vi "getRobotModelStateSpace.vi"(8 "error in (no error)":errorcluster, 10 "StateSpaceTestParameters":T1, 11 "Game in":refnum<class "Game.lvclass">) -> (0 "error out":errorcluster, 1 "State":T2 {"progress" scale=0.0..100.0}, 2 "TestTeam":refnum<class "Ally.lvclass">, 3 "Game out":refnum<class "Game.lvclass">)   [LabVIEW 2021, in "Game.lvclass"]
uses:
  Game.lvclass
  Controls/RobotModelTestState.ctl
  Ally_class/Ally.lvclass
  D:/RoboIme/controle/SSL_AI/Team_class/Team.lvclass
  Game.lvclass/Game.ctl
  Team_class/Team.lvclass/Team.ctl
  Robot_class/Robot.lvclass/Robot.ctl
  <vilib>/Analysis/coordinate.llb/2D Cartesian Coordinate Rotation (Scalar).vi
  Read TestTeam.vi
  Read AllyRef.vi
  Team_class/Read RobotRef.vi
  Robot_class/Read orientation.vi
  Robot_class/Write v_tang.vi
  Robot_class/Write v_norm.vi
  Robot_class/Write v_ang.vi
  Team_class/Write RobotRef.vi
  Robot_class/Robot.lvclass
  Utilities_class/Utilities.lvclass
  <vilib>/Analysis/NI_AALPro.lvlib
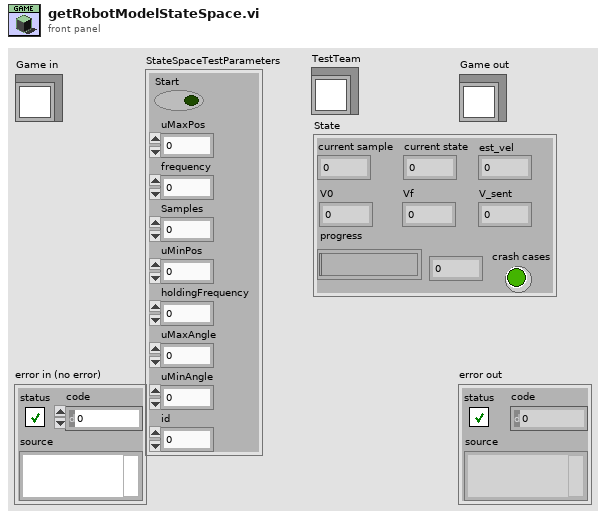
[diagram p1: front panel]
types:
  T1 = cluster{"Start":bool, "uMaxPos":dbl, "frequency":i32, "Samples":dbl, "uMinPos":dbl, "holdingFrequency":dbl, "uMaxAngle":dbl, "uMinAngle":dbl, "id":dbl}
  T2 = typedef "RobotModelTestState.ctl" = cluster{"current sample":i32, "V0":dbl, "Vf":dbl, "progress":dbl, "current state":i32, "est_vel":dbl, "V_sent":dbl, "crash cases":bool}
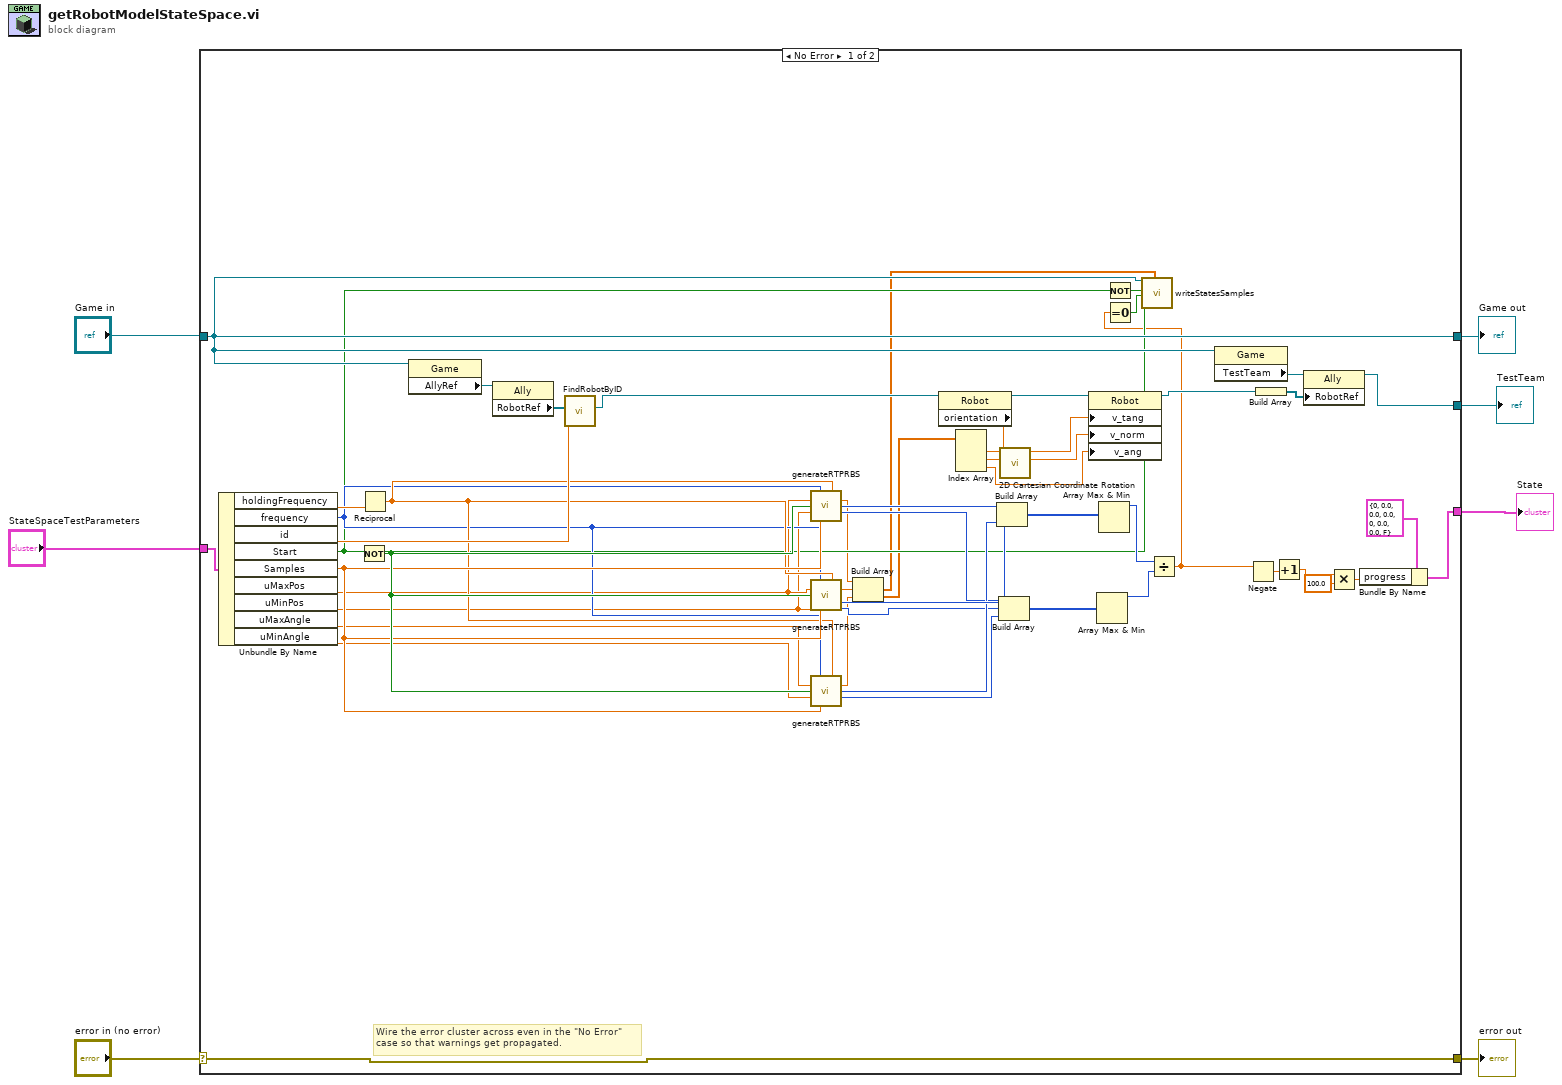
[diagram p0: block diagram]
diagram:
  n1 = case shown="No Error" "error in (no error)" {
    selector: "error in (no error)" -> [w58 w60]
    tunnel: [w58 w60] -> w6
    tunnel: [w21 w59] -> w4
    tunnel: "Game in" -> [w21 w59]
    tunnel: "StateSpaceTestParameters" -> [w55 _]
    tunnel: [w51 _] -> w3
    tunnel: [w49 _] -> w2
    frame No Error {
      # "Wire the error cluster across even in the \"No Error\"\ncase so that warnings get propagated."
      n2 = Unbundle By Name(w55) -> ("holdingFrequency"=w42:dbl, "frequency"=w40:i32, "id"=w54:dbl, "Start"=w19:bool, "Samples"=w43:dbl, "uMaxPos"=w39:dbl, "uMinPos"=w38:dbl, "uMaxAngle"=w37:dbl, "uMinAngle"=w36:dbl)
      n3 = Not(x=w19) -> (.not. x?=w44:bool)
      n4 = Reciprocal(x=w42) -> (1/x=w41:dbl)
      n5 = property class="Game"(reference=w21) -> ("AllyRef"=w57:refnum<class "Ally.lvclass">)  [unwired: 1 in, 2 out]
      n6 = property class="Ally"(reference=w57) -> ("RobotRef"=w56:refnum<class "Robot.lvclass">[])  [unwired: 1 in, 2 out]
      n7 = call "FindRobotByID.vi"("id"=w54, "RobotRef"=w56) -> ("Robot"=w48:refnum<class "Robot.lvclass">)  [unwired: 6 in, 3 out]
      n8 = call "generateRTPRBS.vi"("W"=w40, "Th"=w41, "MAX"=w39, "activate"=w44, "MIN"=w38, "PRBS samples"=w43) -> ("Val"=w18:dbl, "Size"=w35:i32, "totalSize"=w32:i32)  [unwired: 5 in, 2 out]
      n9 = call "generateRTPRBS.vi"("W"=w40, "Th"=w41, "MAX"=w39, "activate"=w44, "MIN"=w38, "PRBS samples"=w43) -> ("Val"=w17:dbl, "Size"=w34:i32, "totalSize"=w31:i32)  [unwired: 5 in, 2 out]
      n10 = call "generateRTPRBS.vi"("W"=w40, "Th"=w41, "MAX"=w37, "activate"=w44, "MIN"=w36, "PRBS samples"=w43) -> ("Val"=w16:dbl, "Size"=w33:i32, "totalSize"=w30:i32)  [unwired: 5 in, 2 out]
      n11 = Build Array(w18, w17, w16) -> (w10:dbl[])
      n12 = property class="Robot"(reference=w48) -> (reference out=w46:refnum<class "Robot.lvclass">, "orientation"=w47:dbl)  [unwired: 1 in, 1 out]
      n13 = Index Array(array=w10) -> (element #1=w15:dbl, element #2=w14:dbl, element #3=w13:dbl)  [unwired: 3 in]
      n14 = Build Array(w35, w34, w33) -> (w29:i32[])
      n15 = Build Array(w32, w31, w30) -> (w28:i32[])
      n16 = call-poly <vilib>:"2D Cartesian Coordinate Rotation.vi"("theta"=w47, "y"=w14, "x"=w15) -> ("y out"=w11:dbl, "x out"=w12:dbl)  [unwired: 6 in, 1 out]
      n17 = property class="Robot"(reference=w46, "v_tang"=w12, "v_norm"=w11, "v_ang"=w13) -> (reference out=w45:refnum<class "Robot.lvclass">)  [unwired: 1 in, 1 out]
      n18 = Array Max & Min(array=w28) -> (max value=w26:i32)  [unwired: 3 out]
      n19 = Array Max & Min(array=w29) -> (max value=w27:i32)  [unwired: 3 out]
      n20 = Not(x=w19) -> (.not. x?=w20:bool)
      n21 = Divide(x=w27, y=w26) -> (x/y=w9:dbl)
      n22 = Equal To 0?(x=w9) -> (x = 0?=w8:bool)
      n23 = call "writeStatesSamples.vi"("Game in"=w21, "Start Recording"=w19, "Clear"=w20, "Dump"=w8, "uk"=w10) -> ()  [unwired: 13 in, 2 out]
      n24 = property class="Game"(reference=w21) -> ("TestTeam"=w53:refnum<class "Ally.lvclass">)  [unwired: 1 in, 2 out]
      n25 = Negate(x=w9) -> (-x=w25:dbl)
      n26 = Build Array(w45) -> (w52:refnum<class "Robot.lvclass">[])
      n27 = Increment(x=w25) -> (x+1=w23:dbl)
      n28 = property class="Ally"(reference=w53, "RobotRef"=w52) -> (reference out=w51:refnum<class "Ally.lvclass">)  [unwired: 1 in, 1 out]
      n29 = Multiply(x=w23, y=100.0) -> (x*y=w22:dbl)
      n30 = Bundle By Name(cluster=T2 {"current sample"=0, "V0"=0.0, "Vf"=0.0, "progress"=0.0, "current state"=0, "est_vel"=0.0, "V_sent"=0.0, "crash cases"=FALSE} ("State 2"), "progress"=w22) -> (w49:T2)
    }
    frame Error {
    }
  }
  "error out" <- w6
  "Game out" <- w4
  "State" <- w2
  "TestTeam" <- w3
